vi "Get Cluster Info.vi"(8 "error in (no error)":errorcluster, 11 "Cluster":variant) -> (0 "error out":errorcluster, 1 "Cluster Name":string, 2 "Values":variant[](array[variant]), 3 "Item Names":string[](array[string]), 4 "HasTypedef":bool, 5 "# Items":i16)   [LabVIEW 2011]
doc: "Get all relevant info about the cluster passed in.\n\n\nVersion 1.0 - 2/14/2013\n\nPhaeron, Inc.\nwww.phaeron.com\ninfo@phaeron.com"
uses:
  <vilib>/Utility/VariantDataType/VariantType.lvlib
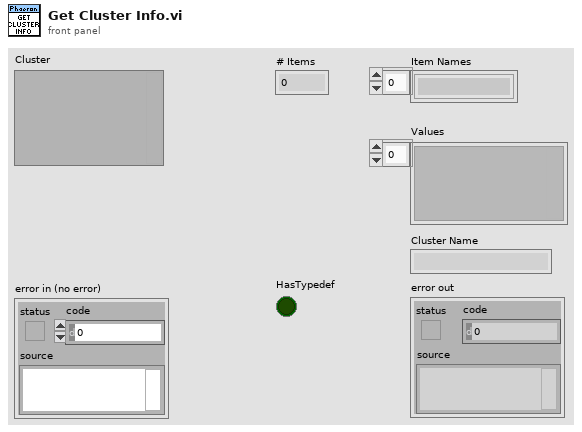
[diagram p1: front panel]
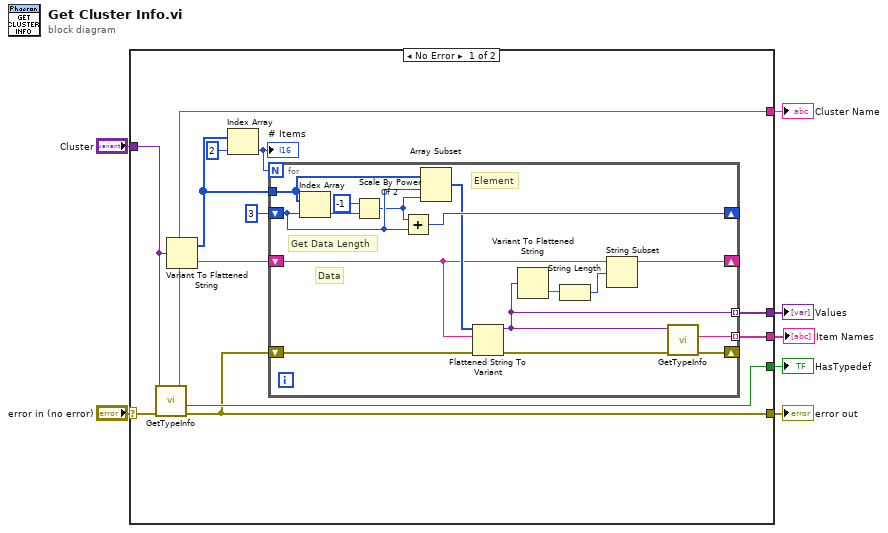
[diagram p0: block diagram]
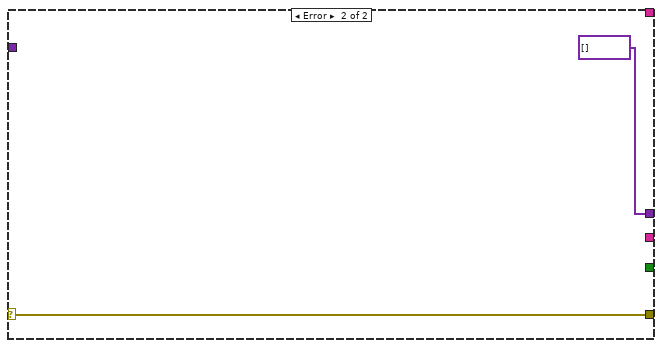
[diagram p2: hidden frame]
diagram:
  n1 = case shown="No Error" "error in (no error)" {
    selector: "error in (no error)" -> [w18 w37]
    tunnel: [w10 w37] -> w6
    tunnel: "Cluster" -> [w16 _]
    tunnel: [w8 variant[] []] -> w4
    tunnel: [w19 _] -> w3
    tunnel: [w17 _] -> w2
    tunnel: [w9 _] -> w1
    frame No Error {
      n2 = call <vilib>:"GetTypeInfo.vi"("error in (no error)"=w18, "Variant"=w16) -> ("error out"=w10:errorcluster, "HasTypedef"=w17:bool, "Name"=w19:string)  [unwired: 5 in, 2 out]
      n3 = Variant To Flattened String(Variant=w16) -> (data string=w14:string, 1:w12:i16[])
      n4 = Index Array(array=w12, index=2) -> (element=w15:i16)
      "# Items" <- w15
      n5 = for {
        N: w15 -> [_]
        shift-right: [w22] -> _
        shift-left: w14 -> [w28]
        tunnel: w12 -> [w32]
        shift-right: [w33] -> _
        shift-left: 3 ("index") -> [w31]
        shift-right: [w25] -> _
        shift-left: w10 -> [w27]
        tunnel: [w24] -> w9 mode=indexing
        tunnel: [w20] -> w8 mode=indexing
        # "Data"
        # "Element"
        # "Get Data Length"
        n6 = Index Array(array=w32, index=w31) -> (element=w34:i16)
        n7 = Scale By Power Of 2(n=i16 -1, x=w34) -> (x*2^n=w30:i16)
        n8 = Add(x=w30, y=w31) -> (x+y=w33:i32)
        n9 = Array Subset(array=w32, index=w31, length=w30) -> (w29:i16[])
        n10 = Flattened String To Variant(4:w27, 6:w28, 7:w29) -> (0:w26:errorcluster, 3:w20:variant)
        n11 = Variant To Flattened String(Variant=w20) -> (data string=w23:string)  [unwired: 1 out]
        n12 = String Length(string=w23) -> (length=w21:i32)
        n13 = String Subset(string=w28, offset (0)=w21) -> (substring=w22:string)  [unwired: 1 in]
        n14 = call <vilib>:"GetTypeInfo.vi"("error in (no error)"=w26, "Variant"=w20) -> ("error out"=w25:errorcluster, "Name"=w24:string)  [unwired: 5 in, 3 out]
      }
    }
    frame Error {
    }
  }
  "error out" <- w6
  "Values" <- w4
  "Cluster Name" <- w3
  "HasTypedef" <- w2
  "Item Names" <- w1
